vi "CosA_FFT.vi"(1 "Rk":dbl[](array[numeric])) -> (0 "Xj":dbl[](array[numeric]))   [LabVIEW 2011]
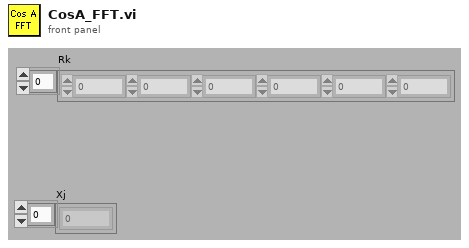
[diagram p1: front panel]
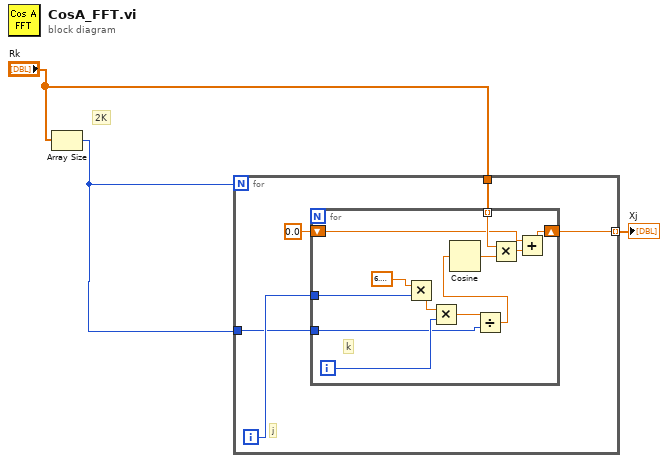
[diagram p0: block diagram]
diagram:
  # "2K"
  n1 = Array Size(array="Rk") -> (size(s)=w1:i32)
  n2 = for {
    N: w1 -> [_]
    tunnel: w1 -> [w7]
    tunnel: "Rk" -> [w6]
    tunnel: [w4] -> w2 mode=indexing
    i -> [w8]
    # "j"
    n3 = for {
      tunnel: w8 -> [w19]
      tunnel: w7 -> [w15]
      tunnel: w6 -> [w12] mode=indexing
      shift-right: [w11] -> w4
      shift-left: 0.0 -> [w9]
      i -> [w17]
      # "k"
      n4 = Multiply(x=6.283185307179586, y=w19) -> (x*y=w18:dbl)
      n5 = Multiply(x=w18, y=w17) -> (x*y=w16:dbl)
      n6 = Divide(x=w16, y=w15) -> (x/y=w14:dbl)
      n7 = Cosine(x=w14) -> (cos(x)=w13:dbl)
      n8 = Multiply(x=w12, y=w13) -> (x*y=w10:dbl)
      n9 = Add(x=w9, y=w10) -> (x+y=w11:dbl)
    }
  }
  "Xj" <- w2
